vi "Scanner Action-Status Start Scan.vi"(8 "error in (no error)":errorcluster, 10 "Message Data":variant, 11 "Data Cluster in":T1={"Link"={"Connection"=enum."USB", "Host or IP address (TCP/IP)"="", "Port (Serial/USB)"="COM1"}, "VISA resource"="", "Writer Queue"=refnum, "Status"=FALSE}) -> (0 "error out":errorcluster, 3 "Data Cluster out":T1={"Link"={"Connection"=enum."USB", "Host or IP address (TCP/IP)"="", "Port (Serial/USB)"="COM1"}, "VISA resource"="", "Writer Queue"=refnum, "Status"=FALSE})   [LabVIEW 2020, in "Hiden Scanner.lvlib"]
uses:
  Hiden Scanner.lvlib
  Scanner Hardware Configuration.ctl
  support/Message Queue/Message Cluster.ctl
  support/HW Message Cluster.ctl
  support/Message Queue/Message Queue.lvlib
  <instrlib>/Hiden/Hiden MS.lvlib
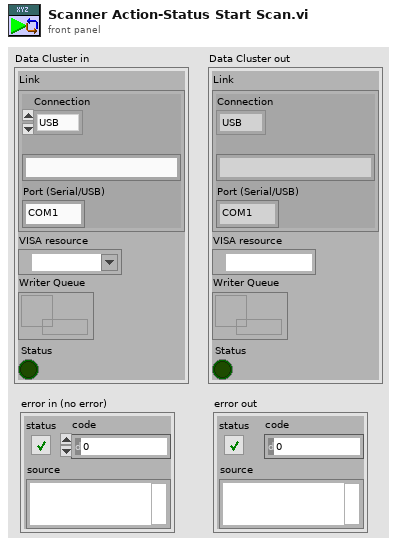
[diagram p1: front panel]
types:
  T1 = typedef "Hiden Scanner.lvlib/Scanner Hardware Configuration.ctl" = cluster{"Link":cluster{"Connection":enum16{"Serial", "TCP/IP", "USB"}, "Host or IP address (TCP/IP)":string, "Port (Serial/USB)":string}, "VISA resource":refnum<visa-resource-name>, "Writer Queue":refnum<queue>, "Status":bool}
  T2 = typedef "Message Queue.lvlib/HW Message Cluster.ctl" = cluster{"Writer Queue":refnum<queue>, "Writer Data":T3}
  T3 = typedef "Message Queue.lvlib/Message Cluster.ctl" = cluster{"Message":string, "Message Data":variant}
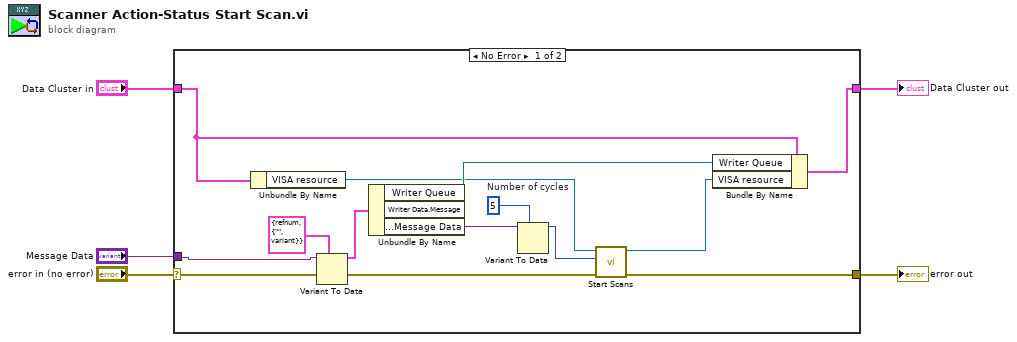
[diagram p0: block diagram]
diagram:
  n1 = case shown="No Error" "error in (no error)" {
    selector: "error in (no error)" -> [w10 w19]
    tunnel: "Message Data" -> [w13 _]
    tunnel: [w14 w20] -> w4
    tunnel: "Data Cluster in" -> [w15 w20]
    tunnel: [w9 w19] -> w2
    frame No Error {
      w7 = u32 5  # Number of cycles
      n2 = Unbundle By Name(w15) -> ("VISA resource"=w12:refnum<visa-resource-name>)
      n3 = Variant To Data(type=T2 {"Writer Queue"=refnum, "Writer Data"={"Message"="", "Message Data"=variant}}, Variant=w13) -> (data=w16:T2)  [unwired: 1 in, 1 out]
      n4 = Unbundle By Name(w16) -> ("Writer Queue"=w17:refnum<queue>, "Writer Data.Message Data"=w8:variant)  [unwired: 1 out]
      n5 = Variant To Data(type=w7, Variant=w8) -> (data=w6:u32)  [unwired: 1 in, 1 out]
      n6 = call <instrlib>:"Start Scans.vi"("error in (no error)"=w10, "Number of cycles (0 = continuous)"=w6, "Connection"=w12) -> ("error out"=w9:errorcluster, "Connection (dup)"=w11:refnum<visa-resource-name>)  [unwired: 5 in, 2 out]
      n7 = Bundle By Name(cluster=w15, "Writer Queue"=w17, "VISA resource"=w11) -> (w14:T1)
    }
    frame Error {
    }
  }
  "Data Cluster out" <- w4
  "error out" <- w2
